vi "Create Paths.vi"(8 "error in (no error)":errorcluster, 11 "Paths":path[](array[path])) -> (0 "error out":errorcluster, 3 "Paths out":path[](array[path]))   [LabVIEW 2017]
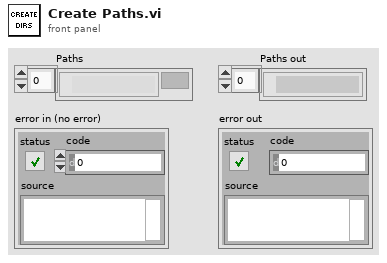
[diagram p1: front panel]
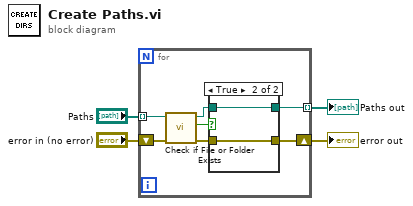
[diagram p0: block diagram]
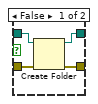
[diagram p2: hidden frame]
diagram:
  n1 = for {
    tunnel: "Paths" -> [w7] mode=indexing
    shift-right: [w10] -> w1
    shift-left: "error in (no error)" -> [w11]
    tunnel: [w9] -> w2 mode=indexing
    n2 = call <vilib>:"Check if File or Folder Exists.vi"("error in (no error)"=w11, "path"=w7) -> ("error out"=w8:errorcluster, "file or folder exists?"=w5:bool, "dup path"=w6:path)  [unwired: 7 in]
    n3 = case shown="True" w5 {
      tunnel: [w15 w16] -> w10
      tunnel: [w14 w17] -> w9
      tunnel: w8 -> [w13 w16]
      tunnel: w6 -> [w12 w17]
      frame False {
        n4 = Create Folder(path (use dialog)=w12, error in=w13) -> (created path=w14:path, error out=w15:errorcluster)  [unwired: 1 in, 1 out]
      }
      frame True {
      }
    }
  }
  "Paths out" <- w2
  "error out" <- w1
